vi "Load Config.vi"(8 "error in (no error)":errorcluster, 11 "Historian Logger in":refnum<class "Historian Logger.lvclass">) -> (0 "error out":errorcluster, 3 "Historian Logger out":refnum<class "Historian Logger.lvclass">)   [LabVIEW 2020, in "VolatusHistorian.lvlib" / "Historian Logger.lvclass"]
uses:
  Historian Logger.lvclass
  C:/dev/lv20CE/relink/lv-volatus/Volatus/Module/Module.lvclass
  Volatus/Module/Module.lvclass/Module.ctl
  VolatusConfig/VolatusConfigElement/VolatusConfigElement.lvclass/VolatusConfigElement.ctl
  Historian Logger.lvclass/Historian Logger.ctl
  Volatus/Module/Config.vi
  VolatusConfig/VolatusConfigElement/Element.vi
  VolatusConfig/Task/Task Config.lvclass
  C:/dev/lv20CE/relink/lv-volatus/VolatusConfig/VolatusConfigElement/VolatusConfigElement.lvclass
  Volatus/Module/Module.lvclass
  VolatusConfig/VolatusConfigElement/VolatusConfigElement.lvclass
  lv-cdm/CDM-Config/Config Element/Config Element.lvclass
  C:/dev/lv20CE/relink/lv-volatus/VolatusHistorian/Historian Logger/Historian Logger.lvclass
  C:/dev/lv20CE/relink/lv-volatus/VolatusConfig/Task/Task Config.lvclass
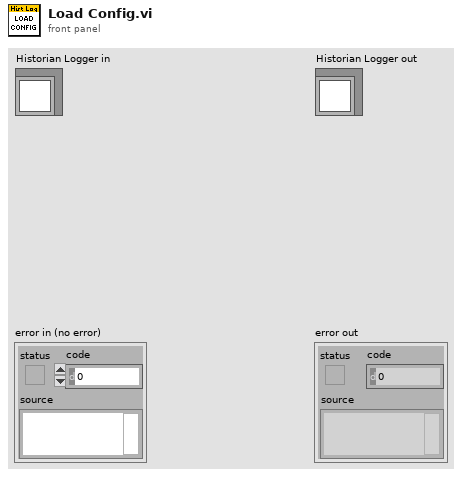
[diagram p1: front panel]
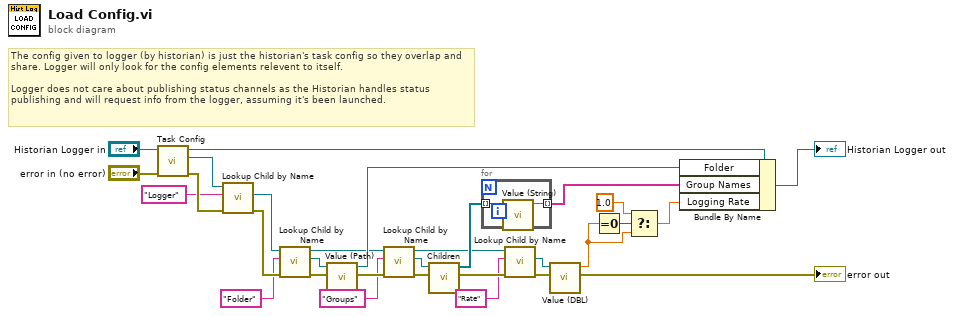
[diagram p0: block diagram]
diagram:
  # "The config given to logger (by historian) is just the historian's task config so they overlap and share. Logger will only look for the config elements relevent to itself.\n\nLogger does not care about publishing status channels as the Historian handles status publishing and will request info from the logger, assuming it's been launched."
  n1 = call "Task Config.vi"("error in (no error)"="error in (no error)", "Module in"="Historian Logger in") -> ("error out"=w28:errorcluster, "Task Config"=w24:refnum<class "Task Config.lvclass">, "Module out"=w25:refnum<class "Historian Logger.lvclass">)  [unwired: 7 in]
  n2 = call "Lookup Child by Name.vi"("error in (no error)"=w28, "Child Name"="Logger", "VolatusConfigElement in"=w24) -> ("error out"=w21:errorcluster, "Child"=w22:refnum<class "Config Element.lvclass">)  [unwired: 5 in, 2 out]
  n3 = call "Lookup Child by Name.vi"("error in (no error)"=w21, "Name"="Folder", "Config Element in"=w22) -> ("error out"=w18:errorcluster, "Child"=w19:refnum<class "Config Element.lvclass">, "Config Element out"=w14:refnum<class "Config Element.lvclass">)  [unwired: 5 in, 1 out]
  n4 = call "Value (Path).vi"("error in (no error)"=w18, "Config Element in"=w19) -> ("error out"=w29:errorcluster, "Path Value"=w16:path)  [unwired: 8 in]
  n5 = call "Lookup Child by Name.vi"("error in (no error)"=w29, "Name"="Groups", "Config Element in"=w14) -> ("error out"=w13:errorcluster, "Child"=w12:refnum<class "Config Element.lvclass">, "Config Element out"=w8:refnum<class "Config Element.lvclass">)  [unwired: 5 in, 1 out]
  n6 = call "Children.vi"("error in (no error)"=w13, "Config Element in"=w12) -> ("error out"=w30:errorcluster, "Elements"=w11:refnum<class "Config Element.lvclass">[])  [unwired: 8 in]
  n7 = for {
    tunnel: w11 -> [w32] mode=indexing
    tunnel: [w31] -> w10 mode=indexing
    n8 = call "Value (String).vi"("Config Element in"=w32) -> ("String Value"=w31:string)  [unwired: 9 in, 1 out]
  }
  n9 = call "Lookup Child by Name.vi"("error in (no error)"=w30, "Name"="Rate", "Config Element in"=w8) -> ("error out"=w7:errorcluster, "Child"=w6:refnum<class "Config Element.lvclass">)  [unwired: 5 in, 2 out]
  n10 = call "Value (DBL).vi"("error in (no error)"=w7, "Config Element in"=w6) -> ("error out"=→"error out":errorcluster, "DBL Value"=w2:dbl)  [unwired: 8 in]
  n11 = Equal To 0?(x=w2) -> (x = 0?=w4:bool)
  n12 = Select(t=1.0, s=w4, f=w2) -> (s? t:f=w1:dbl)
  n13 = Bundle By Name(cluster=w25, "Folder"=w16, "Group Names"=w10, "Logging Rate"=w1) -> (→"Historian Logger out":refnum<class "Historian Logger.lvclass">)
